vi "Running_Ch_Average.vi"(4 "Shift In":dbl[](array[numeric]), 5 "History length":i32=10, 6 "Reset Average after Seconds":dbl=120.0, 7 "New Value":dbl) -> (0 "Shift Out":dbl[](array[numeric]), 1 "standard deviation":dbl format="%0.2f", 3 "mean":dbl format="%0.2f")   [LabVIEW 2022 SP3]
uses:
  <vilib>/Analysis/NI_AALBase.lvlib
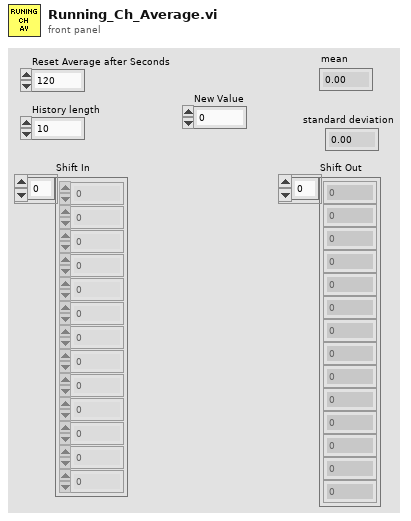
[diagram p1: front panel]
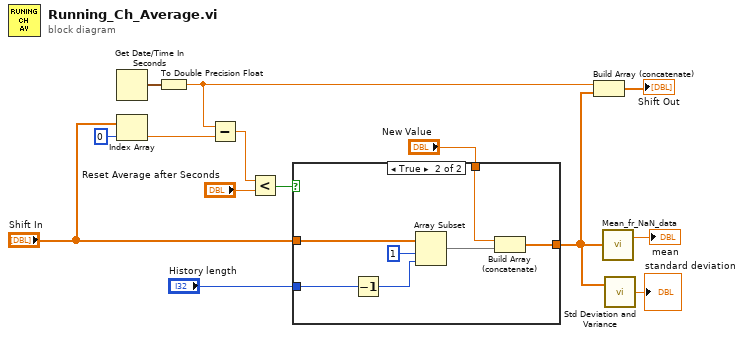
[diagram p0: block diagram]
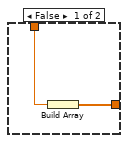
[diagram p2: hidden frame]
diagram:
  n1 = Get Date/Time In Seconds() -> (seconds since 1Jan1904=w13:timestamp)
  n2 = Index Array(array="Shift In", index=0) -> (element=w11:dbl)
  n3 = To Double Precision Float(number=w13) -> (double precision float=w12:dbl)
  n4 = Subtract(x=w12, y=w11) -> (x-y=w10:dbl)
  n5 = Less?(x=w10, y="Reset Average after Seconds") -> (x < y?=w8:bool)
  n6 = case shown="True" w8 {
    tunnel: "Shift In" -> [_ w23]
    tunnel: "New Value" -> [w16 w21]
    tunnel: [w15 w19] -> w2
    tunnel: "History length" -> [_ w18]
    frame False {
      n7 = Build Array(w16) -> (w15:dbl[])
    }
    frame True {
      n8 = Decrement(x=w18) -> (x-1=w17:i32)
      n9 = Array Subset(array=w23, index=1, length=w17) -> (w20:dbl[])
      n10 = Build Array (concatenate)(w21, w20) -> (w19:dbl[])
    }
  }
  n11 = Build Array (concatenate)(w12, w2) -> (→"Shift Out":dbl[])
  n12 = call "Mean_fr_NaN_data.vi"("Data"=w2) -> ("Mean value"=→"mean":dbl)  [unwired: 1 out]
  n13 = call <vilib>:"Std Deviation and Variance.vi"("X"=w2) -> ("standard deviation"=→"standard deviation":dbl)  [unwired: 1 in, 2 out]
